vi "Write DriveMotorReferences.vi"(8 "error in (no error)":errorcluster, 10 "DriveMotorReferences":T1[](array[typedef]), 11 "DriveMotors in":refnum<class "DriveMotors.lvclass">) -> (0 "error out":errorcluster, 3 "DriveMotors out":refnum<class "DriveMotors.lvclass">)   [LabVIEW 2013, in "DriveMotors.lvclass"]
uses:
  DriveMotors.lvclass
  <vilib>/Rock Robotics/WPI/MotorControl/WPI_MotorControlDeviceRef.ctl
  <vilib>/Rock Robotics/SystemInterfaces/Typedef/FPGA_TypedefDigitalModule.ctl
  <vilib>/Rock Robotics/SystemInterfaces/DIO/FPGA_DIOPWMChannel.ctl
  <vilib>/Rock Robotics/WPI/PWM/WPI_PWMDeadband.ctl
  <vilib>/Rock Robotics/WPI/CAN/Jaguar/SubVIs/WPI_CANJaguar_ControlMode.ctl
  <vilib>/Rock Robotics/WPI/PWM/WPI_PWMTransform_ConPane.ctl
  DriveMotors.lvclass/DriveMotors.ctl
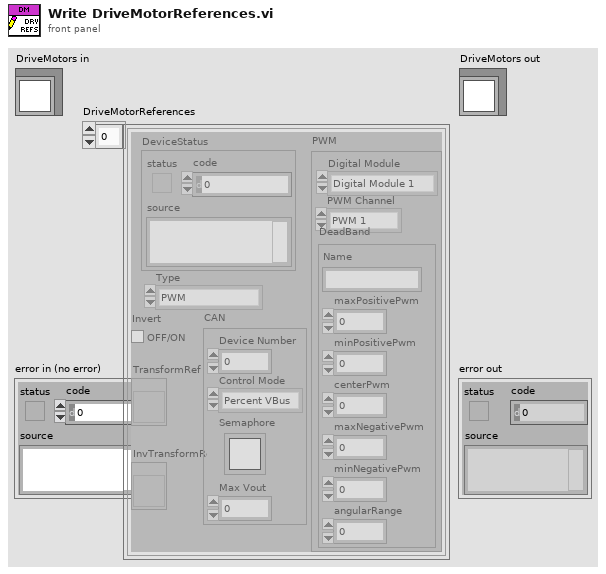
[diagram p1: front panel]
types:
  T1 = typedef "WPI_MotorControlDeviceRef.ctl" = cluster{"DeviceStatus":errorcluster, "Type":enum16{"PWM", "CAN"}, "PWM":cluster{"Digital Module":T2, "PWM Channel":T3, "DeadBand":T4}, "CAN":cluster{"Device Number":u8, "Control Mode":T5, "Semaphore":T6, "Max Vout":dbl}, "Invert":bool, "TransformRef":T7, "InvTransformRef":T7}
  T2 = typedef "FPGA_TypedefDigitalModule.ctl" = enum16{"Digital Module 1", "Digital Module 2"}
  T3 = typedef "FPGA_DIOPWMChannel.ctl" = enum8{"PWM 1", "PWM 2", "PWM 3", "PWM 4", "PWM 5", "PWM 6", "PWM 7", "PWM 8", "PWM 9", "PWM 10", "Invalid"}
  T4 = typedef "WPI_PWMDeadband.ctl" = cluster{"Name":string, "maxPositivePwm":i32, "minPositivePwm":i32, "centerPwm":i32, "maxNegativePwm":i32, "minNegativePwm":i32, "angularRange":u16}
  T5 = typedef "WPI_CANJaguar_ControlMode.ctl" = enum8{"Percent VBus", "Current", "Speed", "Position", "Voltage"}
  T6 = typedef "Semaphore RefNum" = refnum<k1>
  T7 = typedef "WPI_PWMTransform_ConPane.ctl" = refnum<vi>
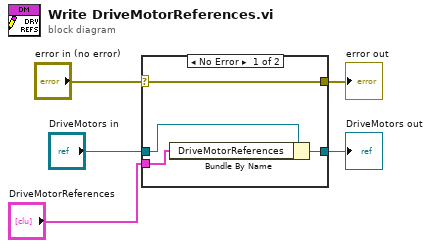
[diagram p0: block diagram]
diagram:
  n1 = case shown="No Error" "error in (no error)" {
    selector: "error in (no error)" -> [w9 w10]
    tunnel: [w9 w10] -> w4
    tunnel: [w7 w11] -> w2
    tunnel: "DriveMotors in" -> [w8 w11]
    tunnel: "DriveMotorReferences" -> [w6 _]
    frame No Error {
      n2 = Bundle By Name(cluster=w8, "DriveMotorReferences"=w6) -> (w7:refnum<class "DriveMotors.lvclass">)
    }
    frame Error {
    }
  }
  "error out" <- w4
  "DriveMotors out" <- w2
